vi "Relay Control - Execute Command.vi"(8 "error in (no error)":errorcluster, 10 "Command":refnum<k21>, 11 "SLSC Switch in":refnum<class "SLSC Switch.lvclass">) -> (0 "error out":errorcluster, 3 "SLSC Switch out":refnum<class "SLSC Switch.lvclass">)   [LabVIEW 2015, in "SLSC Switch.lvclass"]
uses:
  SLSC Switch.lvclass
  SLSC Switch.lvclass/SLSC Switch.ctl
  <vilib>/SLSC/Execute Device Command.vi
  <vilib>/SLSC/SLSC.lvlib
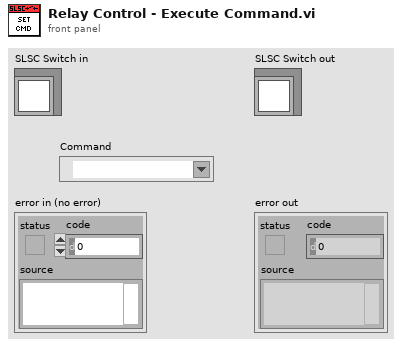
[diagram p1: front panel]
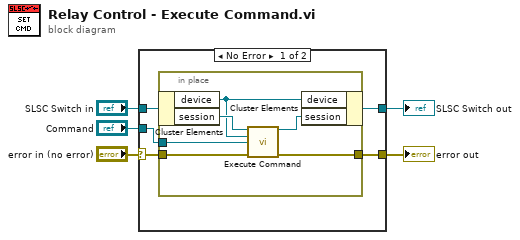
[diagram p0: block diagram]
diagram:
  n1 = case shown="No Error" "error in (no error)" {
    selector: "error in (no error)" -> [w7 w18]
    tunnel: [w10 w18] -> w4
    tunnel: [w9 w17] -> w2
    tunnel: "SLSC Switch in" -> [w8 w17]
    tunnel: "Command" -> [w6 _]
    frame No Error {
      n2 = in-place {
        in-place-border: [w16] -> w10
        in-place-border: w7 -> [w15]
        in-place-border: w6 -> [w12]
        n3 = in-place-cluster #1(w8) -> ("device"=w13:refnum<k21>, "session"=w14:refnum<k21>)
        n4 = call-poly <vilib>:"Execute Command.vi"("session in"=w14, "devices"=w13, "command"=w12, "error in (no error)"=w15) -> ("session out"=w11:refnum<k21>, "error out"=w16:errorcluster)  [unwired: 10 in]
        n5 = in-place-cluster #1("device"=w13, "session"=w11) -> (w9:refnum<class "SLSC Switch.lvclass">)
      }
    }
    frame Error {
    }
  }
  "error out" <- w4
  "SLSC Switch out" <- w2
